vi "beta-2.0.0.vi"() -> ()   [LabVIEW 2016]
uses:
  <vilib>/FPGAPlugInAG/cRIO-9063/niLvFpga_Open_cRIO-9063.vi
  <vilib>/rvi/interface/common/dynamic/niFpgaDynamicAddResources.vi
  <vilib>/Utility/error.llb/Error Cluster From Error Code.vi
  <vilib>/rvi/errors/niLvFpgaAdjustHostInterfaceError.vi
  <vilib>/FPGAPlugInAG/Dynamic/niLvFpga_Close_Dynamic.vi
  <vilib>/rvi/interface/nirviOpenFPGA/nirviOpenFPGA.xnode
  FPGA Bitfiles/multi-functionpr_FPGATarget_multi-function-f_bsn-gyeHrfY.lvbitx
  <vilib>/rvi/interface/nirviReadWriteControl/nirviReadWriteControl.xnode
  <vilib>/rvi/interface/nirviCloseFPGA/nirviCloseFPGA.xnode
  NiFpgaLv.dll
  <vilib>/rvi/interface/Simulation/niFpgaSimulationCallBeginRW.vi
panel:
  in  "OUT15":T1(ring)
  in  "step15":dbl=1.0 format="%#_13g"
  in  "begin15":dbl format="%#_13g"
  in  "end15":dbl=5.0 format="%#_13g"
  in  "OUT14":T1(ring)
  in  "step14":dbl=1.0 format="%#_13g"
  in  "begin14":dbl format="%#_13g"
  in  "end14":dbl=5.0 format="%#_13g"
  in  "OUT13":T1(ring)
  in  "step13":dbl=1.0 format="%#_13g"
  in  "begin13":dbl format="%#_13g"
  in  "end13":dbl=5.0 format="%#_13g"
  in  "OUT12":T1(ring)
  in  "step12":dbl=1.0 format="%#_13g"
  in  "begin12":dbl format="%#_13g"
  in  "end12":dbl=5.0 format="%#_13g"
  in  "OUT11":T1(ring)
  in  "step11":dbl=1.0 format="%#_13g"
  in  "begin11":dbl format="%#_13g"
  in  "end11":dbl=5.0 format="%#_13g"
  in  "OUT10":T1(ring)
  in  "step10":dbl=1.0 format="%#_13g"
  in  "begin10":dbl format="%#_13g"
  in  "end10":dbl=5.0 format="%#_13g"
  in  "OUT9":T1(ring)
  in  "step9":dbl=1.0 format="%#_13g"
  in  "begin9":dbl format="%#_13g"
  in  "end9":dbl=5.0 format="%#_13g"
  in  "OUT8":T1(ring)
  in  "step8":dbl=1.0 format="%#_13g"
  in  "begin8":dbl format="%#_13g"
  in  "end8":dbl=5.0 format="%#_13g"
  in  "OUT7":T1(ring)
  in  "step7":dbl=1.0 format="%#_13g"
  in  "begin7":dbl format="%#_13g"
  in  "end7":dbl=5.0 format="%#_13g"
  in  "OUT6":T1(ring)
  in  "step6":dbl=1.0 format="%#_13g"
  in  "begin6":dbl format="%#_13g"
  in  "end6":dbl=5.0 format="%#_13g"
  in  "OUT5":T1(ring)
  in  "step5":dbl=1.0 format="%#_13g"
  in  "begin5":dbl format="%#_13g"
  in  "end5":dbl=5.0 format="%#_13g"
  in  "OUT4":T1(ring)
  in  "step4":dbl=1.0 format="%#_13g"
  in  "begin4":dbl format="%#_13g"
  in  "end4":dbl=5.0 format="%#_13g"
  in  "OUT3":T1(ring)
  in  "step3":dbl=1.0 format="%#_13g"
  in  "begin3":dbl format="%#_13g"
  in  "end3":dbl=5.0 format="%#_13g"
  in  "OUT2":T1(ring)
  in  "step2":dbl=1.0 format="%#_13g"
  in  "begin2":dbl format="%#_13g"
  in  "end2":dbl=5.0 format="%#_13g"
  in  "OUT1":T1(ring)
  in  "step1":dbl=1.0 format="%#_13g"
  in  "begin1":dbl format="%#_13g"
  in  "end1":dbl=5.0 format="%#_13g"
  in  "end0":dbl=5.0 format="%#_13g"
  in  "begin0":dbl format="%#_13g"
  in  "step0":dbl=1.0 format="%#_13g"
  in  "OUT0":T1(ring)
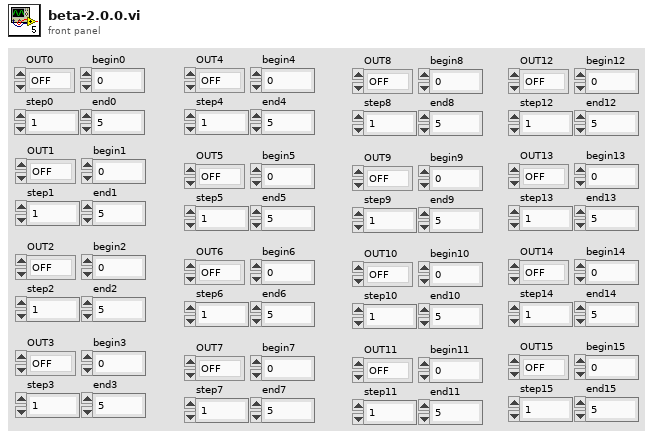
[diagram p1: front panel]
types:
  T1 = enum16{"OFF", "SWITCH", "AND GATE", "OR GATE", "ITERATION"}
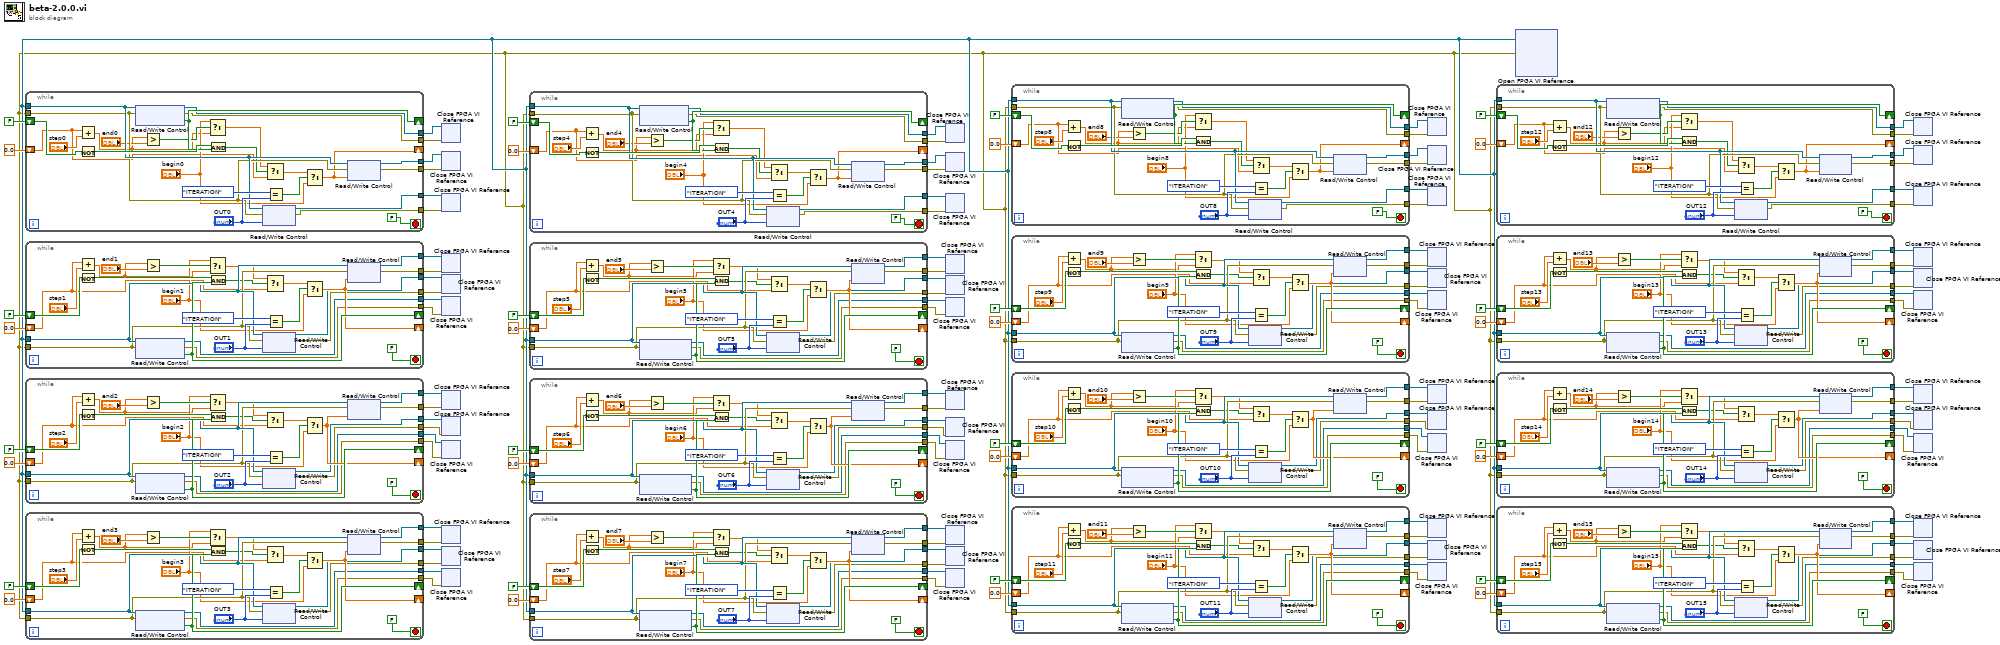
[diagram p0: block diagram]
diagram:
  n1 = xnode "Open FPGA VI Reference"() -> ("FPGA VI Reference Out"=w2:refnum<k20>, "error out"=w1:errorcluster)  [unwired: 2 in]
  n2 = while {
    tunnel: w2 -> [w149]
    tunnel: w1 -> [w148]
    shift-right: [w151] -> _
    shift-left: FALSE -> [w153]
    shift-right: [w146] -> _
    shift-left: 0.0 -> [w138]
    tunnel: [w136] -> w128
    tunnel: [w135] -> w127
    tunnel: [w134] -> w126
    tunnel: [w133] -> w125
    tunnel: [w132] -> w124
    tunnel: [w131] -> w123
    stop <- FALSE stop-if-true
    n3 = Add(x=w138, y="step0") -> (x+y=w140:dbl)
    n4 = Not(x=w153) -> (.not. x?=w152:bool)
    n5 = xnode "Read/Write Control"("FPGA VI Reference In"=w149, "error in"=w148) -> ("FPGA VI Reference Out"=w136:refnum<k20>, "error out"=w135:errorcluster, "Mod2/DIO0"=w151:bool)
    n6 = Greater?(x=w140, y="end0") -> (0:w142:bool)
    n7 = Select(t="begin0", s=w142, f=w140) -> (s? t:f=w139:dbl)
    n8 = And(x=w152, y=w151) -> (x .and. y?=w144:bool)
    n9 = xnode "Read/Write Control"("FPGA VI Reference In"=w149, "error in"=w148, "OUT0"="OUT0") -> ("FPGA VI Reference Out"=w134:refnum<k20>, "error out"=w133:errorcluster)
    n10 = Select(t=w139, s=w144, f=w138) -> (s? t:f=w137:dbl)
    n11 = Equal?(x=T1."ITERATION" ("OUT0"), y="OUT0") -> (x = y?=w147:bool)
    n12 = Select(t=w137, s=w147, f="begin0") -> (s? t:f=w146:dbl)
    n13 = xnode "Read/Write Control"("FPGA VI Reference In"=w149, "error in"=w148, "iter0"=w146) -> ("FPGA VI Reference Out"=w132:refnum<k20>, "error out"=w131:errorcluster)
  }
  n14 = while {
    tunnel: w2 -> [w174]
    tunnel: w1 -> [w173]
    shift-right: [w176] -> _
    shift-left: FALSE -> [w178]
    shift-right: [w171] -> _
    shift-left: 0.0 -> [w163]
    tunnel: [w161] -> w120
    tunnel: [w160] -> w119
    tunnel: [w159] -> w118
    tunnel: [w158] -> w117
    tunnel: [w157] -> w116
    tunnel: [w156] -> w115
    stop <- FALSE stop-if-true
    n15 = Add(x=w163, y="step1") -> (x+y=w165:dbl)
    n16 = Not(x=w178) -> (.not. x?=w177:bool)
    n17 = xnode "Read/Write Control"("FPGA VI Reference In"=w174, "error in"=w173) -> ("FPGA VI Reference Out"=w161:refnum<k20>, "error out"=w160:errorcluster, "Mod2/DIO2"=w176:bool)
    n18 = Greater?(x=w165, y="end1") -> (0:w167:bool)
    n19 = Select(t="begin1", s=w167, f=w165) -> (s? t:f=w164:dbl)
    n20 = And(x=w177, y=w176) -> (x .and. y?=w169:bool)
    n21 = xnode "Read/Write Control"("FPGA VI Reference In"=w174, "error in"=w173, "OUT1"="OUT1") -> ("FPGA VI Reference Out"=w159:refnum<k20>, "error out"=w158:errorcluster)
    n22 = Select(t=w164, s=w169, f=w163) -> (s? t:f=w162:dbl)
    n23 = Equal?(x=T1."ITERATION" ("OUT0"), y="OUT1") -> (x = y?=w172:bool)
    n24 = Select(t=w162, s=w172, f="begin1") -> (s? t:f=w171:dbl)
    n25 = xnode "Read/Write Control"("FPGA VI Reference In"=w174, "error in"=w173, "iter1"=w171) -> ("FPGA VI Reference Out"=w157:refnum<k20>, "error out"=w156:errorcluster)
  }
  n26 = while {
    tunnel: w2 -> [w199]
    tunnel: w1 -> [w198]
    shift-right: [w201] -> _
    shift-left: FALSE -> [w203]
    shift-right: [w196] -> _
    shift-left: 0.0 -> [w188]
    tunnel: [w186] -> w112
    tunnel: [w185] -> w111
    tunnel: [w184] -> w110
    tunnel: [w183] -> w109
    tunnel: [w182] -> w108
    tunnel: [w181] -> w107
    stop <- FALSE stop-if-true
    n27 = Add(x=w188, y="step2") -> (x+y=w190:dbl)
    n28 = Not(x=w203) -> (.not. x?=w202:bool)
    n29 = xnode "Read/Write Control"("FPGA VI Reference In"=w199, "error in"=w198) -> ("FPGA VI Reference Out"=w186:refnum<k20>, "error out"=w185:errorcluster, "Mod2/DIO4"=w201:bool)
    n30 = Greater?(x=w190, y="end2") -> (0:w192:bool)
    n31 = Select(t="begin2", s=w192, f=w190) -> (s? t:f=w189:dbl)
    n32 = And(x=w202, y=w201) -> (x .and. y?=w194:bool)
    n33 = xnode "Read/Write Control"("FPGA VI Reference In"=w199, "error in"=w198, "OUT2"="OUT2") -> ("FPGA VI Reference Out"=w184:refnum<k20>, "error out"=w183:errorcluster)
    n34 = Select(t=w189, s=w194, f=w188) -> (s? t:f=w187:dbl)
    n35 = Equal?(x=T1."ITERATION" ("OUT0"), y="OUT2") -> (x = y?=w197:bool)
    n36 = Select(t=w187, s=w197, f="begin2") -> (s? t:f=w196:dbl)
    n37 = xnode "Read/Write Control"("FPGA VI Reference In"=w199, "error in"=w198, "iter3"=w196) -> ("FPGA VI Reference Out"=w182:refnum<k20>, "error out"=w181:errorcluster)
  }
  n38 = while {
    tunnel: w2 -> [w224]
    tunnel: w1 -> [w223]
    shift-right: [w226] -> _
    shift-left: FALSE -> [w228]
    shift-right: [w221] -> _
    shift-left: 0.0 -> [w213]
    tunnel: [w211] -> w104
    tunnel: [w210] -> w103
    tunnel: [w209] -> w102
    tunnel: [w208] -> w101
    tunnel: [w207] -> w100
    tunnel: [w206] -> w99
    stop <- FALSE stop-if-true
    n39 = Add(x=w213, y="step3") -> (x+y=w215:dbl)
    n40 = Not(x=w228) -> (.not. x?=w227:bool)
    n41 = xnode "Read/Write Control"("FPGA VI Reference In"=w224, "error in"=w223) -> ("FPGA VI Reference Out"=w211:refnum<k20>, "error out"=w210:errorcluster, "Mod2/DIO6"=w226:bool)
    n42 = Greater?(x=w215, y="end3") -> (0:w217:bool)
    n43 = Select(t="begin3", s=w217, f=w215) -> (s? t:f=w214:dbl)
    n44 = And(x=w227, y=w226) -> (x .and. y?=w219:bool)
    n45 = xnode "Read/Write Control"("FPGA VI Reference In"=w224, "error in"=w223, "OUT3"="OUT3") -> ("FPGA VI Reference Out"=w209:refnum<k20>, "error out"=w208:errorcluster)
    n46 = Select(t=w214, s=w219, f=w213) -> (s? t:f=w212:dbl)
    n47 = Equal?(x=T1."ITERATION" ("OUT0"), y="OUT3") -> (x = y?=w222:bool)
    n48 = Select(t=w212, s=w222, f="begin3") -> (s? t:f=w221:dbl)
    n49 = xnode "Read/Write Control"("FPGA VI Reference In"=w224, "error in"=w223, "iter1"=w221) -> ("FPGA VI Reference Out"=w207:refnum<k20>, "error out"=w206:errorcluster)
  }
  n50 = xnode "Close FPGA VI Reference"("FPGA VI Reference In"=w128, "error in"=w127) -> ()  [unwired: 1 out]
  n51 = xnode "Close FPGA VI Reference"("FPGA VI Reference In"=w124, "error in"=w123) -> ()  [unwired: 1 out]
  n52 = xnode "Close FPGA VI Reference"("FPGA VI Reference In"=w126, "error in"=w125) -> ()  [unwired: 1 out]
  n53 = xnode "Close FPGA VI Reference"("FPGA VI Reference In"=w116, "error in"=w115) -> ()  [unwired: 1 out]
  n54 = xnode "Close FPGA VI Reference"("FPGA VI Reference In"=w118, "error in"=w117) -> ()  [unwired: 1 out]
  n55 = xnode "Close FPGA VI Reference"("FPGA VI Reference In"=w120, "error in"=w119) -> ()  [unwired: 1 out]
  n56 = xnode "Close FPGA VI Reference"("FPGA VI Reference In"=w108, "error in"=w107) -> ()  [unwired: 1 out]
  n57 = xnode "Close FPGA VI Reference"("FPGA VI Reference In"=w110, "error in"=w109) -> ()  [unwired: 1 out]
  n58 = xnode "Close FPGA VI Reference"("FPGA VI Reference In"=w112, "error in"=w111) -> ()  [unwired: 1 out]
  n59 = xnode "Close FPGA VI Reference"("FPGA VI Reference In"=w100, "error in"=w99) -> ()  [unwired: 1 out]
  n60 = xnode "Close FPGA VI Reference"("FPGA VI Reference In"=w102, "error in"=w101) -> ()  [unwired: 1 out]
  n61 = xnode "Close FPGA VI Reference"("FPGA VI Reference In"=w104, "error in"=w103) -> ()  [unwired: 1 out]
  n62 = while {
    tunnel: w2 -> [w249]
    tunnel: w1 -> [w248]
    shift-right: [w251] -> _
    shift-left: FALSE -> [w253]
    shift-right: [w246] -> _
    shift-left: 0.0 -> [w238]
    tunnel: [w236] -> w96
    tunnel: [w235] -> w95
    tunnel: [w234] -> w94
    tunnel: [w233] -> w93
    tunnel: [w232] -> w92
    tunnel: [w231] -> w91
    stop <- FALSE stop-if-true
    n63 = Add(x=w238, y="step4") -> (x+y=w240:dbl)
    n64 = Not(x=w253) -> (.not. x?=w252:bool)
    n65 = xnode "Read/Write Control"("FPGA VI Reference In"=w249, "error in"=w248) -> ("FPGA VI Reference Out"=w236:refnum<k20>, "error out"=w235:errorcluster, "Mod2/DIO8"=w251:bool)
    n66 = Greater?(x=w240, y="end4") -> (0:w242:bool)
    n67 = Select(t="begin4", s=w242, f=w240) -> (s? t:f=w239:dbl)
    n68 = And(x=w252, y=w251) -> (x .and. y?=w244:bool)
    n69 = xnode "Read/Write Control"("FPGA VI Reference In"=w249, "error in"=w248, "OUT4"="OUT4") -> ("FPGA VI Reference Out"=w234:refnum<k20>, "error out"=w233:errorcluster)
    n70 = Select(t=w239, s=w244, f=w238) -> (s? t:f=w237:dbl)
    n71 = Equal?(x=T1."ITERATION" ("OUT0"), y="OUT4") -> (x = y?=w247:bool)
    n72 = Select(t=w237, s=w247, f="begin4") -> (s? t:f=w246:dbl)
    n73 = xnode "Read/Write Control"("FPGA VI Reference In"=w249, "error in"=w248, "iter4"=w246) -> ("FPGA VI Reference Out"=w232:refnum<k20>, "error out"=w231:errorcluster)
  }
  n74 = while {
    tunnel: w2 -> [w274]
    tunnel: w1 -> [w273]
    shift-right: [w276] -> _
    shift-left: FALSE -> [w278]
    shift-right: [w271] -> _
    shift-left: 0.0 -> [w263]
    tunnel: [w261] -> w88
    tunnel: [w260] -> w87
    tunnel: [w259] -> w86
    tunnel: [w258] -> w85
    tunnel: [w257] -> w84
    tunnel: [w256] -> w83
    stop <- FALSE stop-if-true
    n75 = Add(x=w263, y="step5") -> (x+y=w265:dbl)
    n76 = Not(x=w278) -> (.not. x?=w277:bool)
    n77 = xnode "Read/Write Control"("FPGA VI Reference In"=w274, "error in"=w273) -> ("FPGA VI Reference Out"=w261:refnum<k20>, "error out"=w260:errorcluster, "Mod2/DIO10"=w276:bool)
    n78 = Greater?(x=w265, y="end5") -> (0:w267:bool)
    n79 = Select(t="begin5", s=w267, f=w265) -> (s? t:f=w264:dbl)
    n80 = And(x=w277, y=w276) -> (x .and. y?=w269:bool)
    n81 = xnode "Read/Write Control"("FPGA VI Reference In"=w274, "error in"=w273, "OUT5"="OUT5") -> ("FPGA VI Reference Out"=w259:refnum<k20>, "error out"=w258:errorcluster)
    n82 = Select(t=w264, s=w269, f=w263) -> (s? t:f=w262:dbl)
    n83 = Equal?(x=T1."ITERATION" ("OUT0"), y="OUT5") -> (x = y?=w272:bool)
    n84 = Select(t=w262, s=w272, f="begin5") -> (s? t:f=w271:dbl)
    n85 = xnode "Read/Write Control"("FPGA VI Reference In"=w274, "error in"=w273, "iter5"=w271) -> ("FPGA VI Reference Out"=w257:refnum<k20>, "error out"=w256:errorcluster)
  }
  n86 = while {
    tunnel: w2 -> [w299]
    tunnel: w1 -> [w298]
    shift-right: [w301] -> _
    shift-left: FALSE -> [w303]
    shift-right: [w296] -> _
    shift-left: 0.0 -> [w288]
    tunnel: [w286] -> w80
    tunnel: [w285] -> w79
    tunnel: [w284] -> w78
    tunnel: [w283] -> w77
    tunnel: [w282] -> w76
    tunnel: [w281] -> w75
    stop <- FALSE stop-if-true
    n87 = Add(x=w288, y="step6") -> (x+y=w290:dbl)
    n88 = Not(x=w303) -> (.not. x?=w302:bool)
    n89 = xnode "Read/Write Control"("FPGA VI Reference In"=w299, "error in"=w298) -> ("FPGA VI Reference Out"=w286:refnum<k20>, "error out"=w285:errorcluster, "Mod2/DIO12"=w301:bool)
    n90 = Greater?(x=w290, y="end6") -> (0:w292:bool)
    n91 = Select(t="begin6", s=w292, f=w290) -> (s? t:f=w289:dbl)
    n92 = And(x=w302, y=w301) -> (x .and. y?=w294:bool)
    n93 = xnode "Read/Write Control"("FPGA VI Reference In"=w299, "error in"=w298, "OUT6"="OUT6") -> ("FPGA VI Reference Out"=w284:refnum<k20>, "error out"=w283:errorcluster)
    n94 = Select(t=w289, s=w294, f=w288) -> (s? t:f=w287:dbl)
    n95 = Equal?(x=T1."ITERATION" ("OUT0"), y="OUT6") -> (x = y?=w297:bool)
    n96 = Select(t=w287, s=w297, f="begin6") -> (s? t:f=w296:dbl)
    n97 = xnode "Read/Write Control"("FPGA VI Reference In"=w299, "error in"=w298, "iter6"=w296) -> ("FPGA VI Reference Out"=w282:refnum<k20>, "error out"=w281:errorcluster)
  }
  n98 = while {
    tunnel: w2 -> [w324]
    tunnel: w1 -> [w323]
    shift-right: [w326] -> _
    shift-left: FALSE -> [w328]
    shift-right: [w321] -> _
    shift-left: 0.0 -> [w313]
    tunnel: [w311] -> w72
    tunnel: [w310] -> w71
    tunnel: [w309] -> w70
    tunnel: [w308] -> w69
    tunnel: [w307] -> w68
    tunnel: [w306] -> w67
    stop <- FALSE stop-if-true
    n99 = Add(x=w313, y="step7") -> (x+y=w315:dbl)
    n100 = Not(x=w328) -> (.not. x?=w327:bool)
    n101 = xnode "Read/Write Control"("FPGA VI Reference In"=w324, "error in"=w323) -> ("FPGA VI Reference Out"=w311:refnum<k20>, "error out"=w310:errorcluster, "Mod2/DIO14"=w326:bool)
    n102 = Greater?(x=w315, y="end7") -> (0:w317:bool)
    n103 = Select(t="begin7", s=w317, f=w315) -> (s? t:f=w314:dbl)
    n104 = And(x=w327, y=w326) -> (x .and. y?=w319:bool)
    n105 = xnode "Read/Write Control"("FPGA VI Reference In"=w324, "error in"=w323, "OUT7"="OUT7") -> ("FPGA VI Reference Out"=w309:refnum<k20>, "error out"=w308:errorcluster)
    n106 = Select(t=w314, s=w319, f=w313) -> (s? t:f=w312:dbl)
    n107 = Equal?(x=T1."ITERATION" ("OUT0"), y="OUT7") -> (x = y?=w322:bool)
    n108 = Select(t=w312, s=w322, f="begin7") -> (s? t:f=w321:dbl)
    n109 = xnode "Read/Write Control"("FPGA VI Reference In"=w324, "error in"=w323, "iter7"=w321) -> ("FPGA VI Reference Out"=w307:refnum<k20>, "error out"=w306:errorcluster)
  }
  n110 = xnode "Close FPGA VI Reference"("FPGA VI Reference In"=w96, "error in"=w95) -> ()  [unwired: 1 out]
  n111 = xnode "Close FPGA VI Reference"("FPGA VI Reference In"=w92, "error in"=w91) -> ()  [unwired: 1 out]
  n112 = xnode "Close FPGA VI Reference"("FPGA VI Reference In"=w94, "error in"=w93) -> ()  [unwired: 1 out]
  n113 = xnode "Close FPGA VI Reference"("FPGA VI Reference In"=w84, "error in"=w83) -> ()  [unwired: 1 out]
  n114 = xnode "Close FPGA VI Reference"("FPGA VI Reference In"=w86, "error in"=w85) -> ()  [unwired: 1 out]
  n115 = xnode "Close FPGA VI Reference"("FPGA VI Reference In"=w88, "error in"=w87) -> ()  [unwired: 1 out]
  n116 = xnode "Close FPGA VI Reference"("FPGA VI Reference In"=w76, "error in"=w75) -> ()  [unwired: 1 out]
  n117 = xnode "Close FPGA VI Reference"("FPGA VI Reference In"=w78, "error in"=w77) -> ()  [unwired: 1 out]
  n118 = xnode "Close FPGA VI Reference"("FPGA VI Reference In"=w80, "error in"=w79) -> ()  [unwired: 1 out]
  n119 = xnode "Close FPGA VI Reference"("FPGA VI Reference In"=w68, "error in"=w67) -> ()  [unwired: 1 out]
  n120 = xnode "Close FPGA VI Reference"("FPGA VI Reference In"=w70, "error in"=w69) -> ()  [unwired: 1 out]
  n121 = xnode "Close FPGA VI Reference"("FPGA VI Reference In"=w72, "error in"=w71) -> ()  [unwired: 1 out]
  n122 = while {
    tunnel: w2 -> [w349]
    tunnel: w1 -> [w348]
    shift-right: [w351] -> _
    shift-left: FALSE -> [w353]
    shift-right: [w346] -> _
    shift-left: 0.0 -> [w338]
    tunnel: [w336] -> w64
    tunnel: [w335] -> w63
    tunnel: [w334] -> w62
    tunnel: [w333] -> w61
    tunnel: [w332] -> w60
    tunnel: [w331] -> w59
    stop <- FALSE stop-if-true
    n123 = Add(x=w338, y="step8") -> (x+y=w340:dbl)
    n124 = Not(x=w353) -> (.not. x?=w352:bool)
    n125 = xnode "Read/Write Control"("FPGA VI Reference In"=w349, "error in"=w348) -> ("FPGA VI Reference Out"=w336:refnum<k20>, "error out"=w335:errorcluster, "Mod2/DIO16"=w351:bool)
    n126 = Greater?(x=w340, y="end8") -> (0:w342:bool)
    n127 = Select(t="begin8", s=w342, f=w340) -> (s? t:f=w339:dbl)
    n128 = And(x=w352, y=w351) -> (x .and. y?=w344:bool)
    n129 = xnode "Read/Write Control"("FPGA VI Reference In"=w349, "error in"=w348, "OUT8"="OUT8") -> ("FPGA VI Reference Out"=w334:refnum<k20>, "error out"=w333:errorcluster)
    n130 = Select(t=w339, s=w344, f=w338) -> (s? t:f=w337:dbl)
    n131 = Equal?(x=T1."ITERATION" ("OUT0"), y="OUT8") -> (x = y?=w347:bool)
    n132 = Select(t=w337, s=w347, f="begin8") -> (s? t:f=w346:dbl)
    n133 = xnode "Read/Write Control"("FPGA VI Reference In"=w349, "error in"=w348, "iter8"=w346) -> ("FPGA VI Reference Out"=w332:refnum<k20>, "error out"=w331:errorcluster)
  }
  n134 = while {
    tunnel: w2 -> [w374]
    tunnel: w1 -> [w373]
    shift-right: [w376] -> _
    shift-left: FALSE -> [w378]
    shift-right: [w371] -> _
    shift-left: 0.0 -> [w363]
    tunnel: [w361] -> w56
    tunnel: [w360] -> w55
    tunnel: [w359] -> w54
    tunnel: [w358] -> w53
    tunnel: [w357] -> w52
    tunnel: [w356] -> w51
    stop <- FALSE stop-if-true
    n135 = Add(x=w363, y="step9") -> (x+y=w365:dbl)
    n136 = Not(x=w378) -> (.not. x?=w377:bool)
    n137 = xnode "Read/Write Control"("FPGA VI Reference In"=w374, "error in"=w373) -> ("FPGA VI Reference Out"=w361:refnum<k20>, "error out"=w360:errorcluster, "Mod2/DIO18"=w376:bool)
    n138 = Greater?(x=w365, y="end9") -> (0:w367:bool)
    n139 = Select(t="begin9", s=w367, f=w365) -> (s? t:f=w364:dbl)
    n140 = And(x=w377, y=w376) -> (x .and. y?=w369:bool)
    n141 = xnode "Read/Write Control"("FPGA VI Reference In"=w374, "error in"=w373, "OUT9"="OUT9") -> ("FPGA VI Reference Out"=w359:refnum<k20>, "error out"=w358:errorcluster)
    n142 = Select(t=w364, s=w369, f=w363) -> (s? t:f=w362:dbl)
    n143 = Equal?(x=T1."ITERATION" ("OUT0"), y="OUT9") -> (x = y?=w372:bool)
    n144 = Select(t=w362, s=w372, f="begin9") -> (s? t:f=w371:dbl)
    n145 = xnode "Read/Write Control"("FPGA VI Reference In"=w374, "error in"=w373, "iter9"=w371) -> ("FPGA VI Reference Out"=w357:refnum<k20>, "error out"=w356:errorcluster)
  }
  n146 = while {
    tunnel: w2 -> [w399]
    tunnel: w1 -> [w398]
    shift-right: [w401] -> _
    shift-left: FALSE -> [w403]
    shift-right: [w396] -> _
    shift-left: 0.0 -> [w388]
    tunnel: [w386] -> w48
    tunnel: [w385] -> w47
    tunnel: [w384] -> w46
    tunnel: [w383] -> w45
    tunnel: [w382] -> w44
    tunnel: [w381] -> w43
    stop <- FALSE stop-if-true
    n147 = Add(x=w388, y="step10") -> (x+y=w390:dbl)
    n148 = Not(x=w403) -> (.not. x?=w402:bool)
    n149 = xnode "Read/Write Control"("FPGA VI Reference In"=w399, "error in"=w398) -> ("FPGA VI Reference Out"=w386:refnum<k20>, "error out"=w385:errorcluster, "Mod2/DIO20"=w401:bool)
    n150 = Greater?(x=w390, y="end10") -> (0:w392:bool)
    n151 = Select(t="begin10", s=w392, f=w390) -> (s? t:f=w389:dbl)
    n152 = And(x=w402, y=w401) -> (x .and. y?=w394:bool)
    n153 = xnode "Read/Write Control"("FPGA VI Reference In"=w399, "error in"=w398, "OUT10"="OUT10") -> ("FPGA VI Reference Out"=w384:refnum<k20>, "error out"=w383:errorcluster)
    n154 = Select(t=w389, s=w394, f=w388) -> (s? t:f=w387:dbl)
    n155 = Equal?(x=T1."ITERATION" ("OUT0"), y="OUT10") -> (x = y?=w397:bool)
    n156 = Select(t=w387, s=w397, f="begin10") -> (s? t:f=w396:dbl)
    n157 = xnode "Read/Write Control"("FPGA VI Reference In"=w399, "error in"=w398, "iter10"=w396) -> ("FPGA VI Reference Out"=w382:refnum<k20>, "error out"=w381:errorcluster)
  }
  n158 = while {
    tunnel: w2 -> [w424]
    tunnel: w1 -> [w423]
    shift-right: [w426] -> _
    shift-left: FALSE -> [w428]
    shift-right: [w421] -> _
    shift-left: 0.0 -> [w413]
    tunnel: [w411] -> w40
    tunnel: [w410] -> w39
    tunnel: [w409] -> w38
    tunnel: [w408] -> w37
    tunnel: [w407] -> w36
    tunnel: [w406] -> w35
    stop <- FALSE stop-if-true
    n159 = Add(x=w413, y="step11") -> (x+y=w415:dbl)
    n160 = Not(x=w428) -> (.not. x?=w427:bool)
    n161 = xnode "Read/Write Control"("FPGA VI Reference In"=w424, "error in"=w423) -> ("FPGA VI Reference Out"=w411:refnum<k20>, "error out"=w410:errorcluster, "Mod2/DIO22"=w426:bool)
    n162 = Greater?(x=w415, y="end11") -> (0:w417:bool)
    n163 = Select(t="begin11", s=w417, f=w415) -> (s? t:f=w414:dbl)
    n164 = And(x=w427, y=w426) -> (x .and. y?=w419:bool)
    n165 = xnode "Read/Write Control"("FPGA VI Reference In"=w424, "error in"=w423, "OUT11"="OUT11") -> ("FPGA VI Reference Out"=w409:refnum<k20>, "error out"=w408:errorcluster)
    n166 = Select(t=w414, s=w419, f=w413) -> (s? t:f=w412:dbl)
    n167 = Equal?(x=T1."ITERATION" ("OUT0"), y="OUT11") -> (x = y?=w422:bool)
    n168 = Select(t=w412, s=w422, f="begin11") -> (s? t:f=w421:dbl)
    n169 = xnode "Read/Write Control"("FPGA VI Reference In"=w424, "error in"=w423, "iter11"=w421) -> ("FPGA VI Reference Out"=w407:refnum<k20>, "error out"=w406:errorcluster)
  }
  n170 = xnode "Close FPGA VI Reference"("FPGA VI Reference In"=w64, "error in"=w63) -> ()  [unwired: 1 out]
  n171 = xnode "Close FPGA VI Reference"("FPGA VI Reference In"=w60, "error in"=w59) -> ()  [unwired: 1 out]
  n172 = xnode "Close FPGA VI Reference"("FPGA VI Reference In"=w62, "error in"=w61) -> ()  [unwired: 1 out]
  n173 = xnode "Close FPGA VI Reference"("FPGA VI Reference In"=w52, "error in"=w51) -> ()  [unwired: 1 out]
  n174 = xnode "Close FPGA VI Reference"("FPGA VI Reference In"=w54, "error in"=w53) -> ()  [unwired: 1 out]
  n175 = xnode "Close FPGA VI Reference"("FPGA VI Reference In"=w56, "error in"=w55) -> ()  [unwired: 1 out]
  n176 = xnode "Close FPGA VI Reference"("FPGA VI Reference In"=w44, "error in"=w43) -> ()  [unwired: 1 out]
  n177 = xnode "Close FPGA VI Reference"("FPGA VI Reference In"=w46, "error in"=w45) -> ()  [unwired: 1 out]
  n178 = xnode "Close FPGA VI Reference"("FPGA VI Reference In"=w48, "error in"=w47) -> ()  [unwired: 1 out]
  n179 = xnode "Close FPGA VI Reference"("FPGA VI Reference In"=w36, "error in"=w35) -> ()  [unwired: 1 out]
  n180 = xnode "Close FPGA VI Reference"("FPGA VI Reference In"=w38, "error in"=w37) -> ()  [unwired: 1 out]
  n181 = xnode "Close FPGA VI Reference"("FPGA VI Reference In"=w40, "error in"=w39) -> ()  [unwired: 1 out]
  n182 = while {
    tunnel: w2 -> [w449]
    tunnel: w1 -> [w448]
    shift-right: [w451] -> _
    shift-left: FALSE -> [w453]
    shift-right: [w446] -> _
    shift-left: 0.0 -> [w438]
    tunnel: [w436] -> w32
    tunnel: [w435] -> w31
    tunnel: [w434] -> w30
    tunnel: [w433] -> w29
    tunnel: [w432] -> w28
    tunnel: [w431] -> w27
    stop <- FALSE stop-if-true
    n183 = Add(x=w438, y="step12") -> (x+y=w440:dbl)
    n184 = Not(x=w453) -> (.not. x?=w452:bool)
    n185 = xnode "Read/Write Control"("FPGA VI Reference In"=w449, "error in"=w448) -> ("FPGA VI Reference Out"=w436:refnum<k20>, "error out"=w435:errorcluster, "Mod2/DIO24"=w451:bool)
    n186 = Greater?(x=w440, y="end12") -> (0:w442:bool)
    n187 = Select(t="begin12", s=w442, f=w440) -> (s? t:f=w439:dbl)
    n188 = And(x=w452, y=w451) -> (x .and. y?=w444:bool)
    n189 = xnode "Read/Write Control"("FPGA VI Reference In"=w449, "error in"=w448, "OUT12"="OUT12") -> ("FPGA VI Reference Out"=w434:refnum<k20>, "error out"=w433:errorcluster)
    n190 = Select(t=w439, s=w444, f=w438) -> (s? t:f=w437:dbl)
    n191 = Equal?(x=T1."ITERATION" ("OUT0"), y="OUT12") -> (x = y?=w447:bool)
    n192 = Select(t=w437, s=w447, f="begin12") -> (s? t:f=w446:dbl)
    n193 = xnode "Read/Write Control"("FPGA VI Reference In"=w449, "error in"=w448, "iter12"=w446) -> ("FPGA VI Reference Out"=w432:refnum<k20>, "error out"=w431:errorcluster)
  }
  n194 = while {
    tunnel: w2 -> [w474]
    tunnel: w1 -> [w473]
    shift-right: [w476] -> _
    shift-left: FALSE -> [w478]
    shift-right: [w471] -> _
    shift-left: 0.0 -> [w463]
    tunnel: [w461] -> w24
    tunnel: [w460] -> w23
    tunnel: [w459] -> w22
    tunnel: [w458] -> w21
    tunnel: [w457] -> w20
    tunnel: [w456] -> w19
    stop <- FALSE stop-if-true
    n195 = Add(x=w463, y="step13") -> (x+y=w465:dbl)
    n196 = Not(x=w478) -> (.not. x?=w477:bool)
    n197 = xnode "Read/Write Control"("FPGA VI Reference In"=w474, "error in"=w473) -> ("FPGA VI Reference Out"=w461:refnum<k20>, "error out"=w460:errorcluster, "Mod2/DIO26"=w476:bool)
    n198 = Greater?(x=w465, y="end13") -> (0:w467:bool)
    n199 = Select(t="begin13", s=w467, f=w465) -> (s? t:f=w464:dbl)
    n200 = And(x=w477, y=w476) -> (x .and. y?=w469:bool)
    n201 = xnode "Read/Write Control"("FPGA VI Reference In"=w474, "error in"=w473, "OUT13"="OUT13") -> ("FPGA VI Reference Out"=w459:refnum<k20>, "error out"=w458:errorcluster)
    n202 = Select(t=w464, s=w469, f=w463) -> (s? t:f=w462:dbl)
    n203 = Equal?(x=T1."ITERATION" ("OUT0"), y="OUT13") -> (x = y?=w472:bool)
    n204 = Select(t=w462, s=w472, f="begin13") -> (s? t:f=w471:dbl)
    n205 = xnode "Read/Write Control"("FPGA VI Reference In"=w474, "error in"=w473, "iter13"=w471) -> ("FPGA VI Reference Out"=w457:refnum<k20>, "error out"=w456:errorcluster)
  }
  n206 = while {
    tunnel: w2 -> [w499]
    tunnel: w1 -> [w498]
    shift-right: [w501] -> _
    shift-left: FALSE -> [w503]
    shift-right: [w496] -> _
    shift-left: 0.0 -> [w488]
    tunnel: [w486] -> w16
    tunnel: [w485] -> w15
    tunnel: [w484] -> w14
    tunnel: [w483] -> w13
    tunnel: [w482] -> w12
    tunnel: [w481] -> w11
    stop <- FALSE stop-if-true
    n207 = Add(x=w488, y="step14") -> (x+y=w490:dbl)
    n208 = Not(x=w503) -> (.not. x?=w502:bool)
    n209 = xnode "Read/Write Control"("FPGA VI Reference In"=w499, "error in"=w498) -> ("FPGA VI Reference Out"=w486:refnum<k20>, "error out"=w485:errorcluster, "Mod2/DIO28"=w501:bool)
    n210 = Greater?(x=w490, y="end14") -> (0:w492:bool)
    n211 = Select(t="begin14", s=w492, f=w490) -> (s? t:f=w489:dbl)
    n212 = And(x=w502, y=w501) -> (x .and. y?=w494:bool)
    n213 = xnode "Read/Write Control"("FPGA VI Reference In"=w499, "error in"=w498, "OUT14"="OUT14") -> ("FPGA VI Reference Out"=w484:refnum<k20>, "error out"=w483:errorcluster)
    n214 = Select(t=w489, s=w494, f=w488) -> (s? t:f=w487:dbl)
    n215 = Equal?(x=T1."ITERATION" ("OUT0"), y="OUT14") -> (x = y?=w497:bool)
    n216 = Select(t=w487, s=w497, f="begin14") -> (s? t:f=w496:dbl)
    n217 = xnode "Read/Write Control"("FPGA VI Reference In"=w499, "error in"=w498, "iter14"=w496) -> ("FPGA VI Reference Out"=w482:refnum<k20>, "error out"=w481:errorcluster)
  }
  n218 = while {
    tunnel: w2 -> [w524]
    tunnel: w1 -> [w523]
    shift-right: [w526] -> _
    shift-left: FALSE -> [w528]
    shift-right: [w521] -> _
    shift-left: 0.0 -> [w513]
    tunnel: [w511] -> w8
    tunnel: [w510] -> w7
    tunnel: [w509] -> w6
    tunnel: [w508] -> w5
    tunnel: [w507] -> w4
    tunnel: [w506] -> w3
    stop <- FALSE stop-if-true
    n219 = Add(x=w513, y="step15") -> (x+y=w515:dbl)
    n220 = Not(x=w528) -> (.not. x?=w527:bool)
    n221 = xnode "Read/Write Control"("FPGA VI Reference In"=w524, "error in"=w523) -> ("FPGA VI Reference Out"=w511:refnum<k20>, "error out"=w510:errorcluster, "Mod2/DIO30"=w526:bool)
    n222 = Greater?(x=w515, y="end15") -> (0:w517:bool)
    n223 = Select(t="begin15", s=w517, f=w515) -> (s? t:f=w514:dbl)
    n224 = And(x=w527, y=w526) -> (x .and. y?=w519:bool)
    n225 = xnode "Read/Write Control"("FPGA VI Reference In"=w524, "error in"=w523, "OUT15"="OUT15") -> ("FPGA VI Reference Out"=w509:refnum<k20>, "error out"=w508:errorcluster)
    n226 = Select(t=w514, s=w519, f=w513) -> (s? t:f=w512:dbl)
    n227 = Equal?(x=T1."ITERATION" ("OUT0"), y="OUT15") -> (x = y?=w522:bool)
    n228 = Select(t=w512, s=w522, f="begin15") -> (s? t:f=w521:dbl)
    n229 = xnode "Read/Write Control"("FPGA VI Reference In"=w524, "error in"=w523, "iter15"=w521) -> ("FPGA VI Reference Out"=w507:refnum<k20>, "error out"=w506:errorcluster)
  }
  n230 = xnode "Close FPGA VI Reference"("FPGA VI Reference In"=w32, "error in"=w31) -> ()  [unwired: 1 out]
  n231 = xnode "Close FPGA VI Reference"("FPGA VI Reference In"=w28, "error in"=w27) -> ()  [unwired: 1 out]
  n232 = xnode "Close FPGA VI Reference"("FPGA VI Reference In"=w30, "error in"=w29) -> ()  [unwired: 1 out]
  n233 = xnode "Close FPGA VI Reference"("FPGA VI Reference In"=w20, "error in"=w19) -> ()  [unwired: 1 out]
  n234 = xnode "Close FPGA VI Reference"("FPGA VI Reference In"=w22, "error in"=w21) -> ()  [unwired: 1 out]
  n235 = xnode "Close FPGA VI Reference"("FPGA VI Reference In"=w24, "error in"=w23) -> ()  [unwired: 1 out]
  n236 = xnode "Close FPGA VI Reference"("FPGA VI Reference In"=w12, "error in"=w11) -> ()  [unwired: 1 out]
  n237 = xnode "Close FPGA VI Reference"("FPGA VI Reference In"=w14, "error in"=w13) -> ()  [unwired: 1 out]
  n238 = xnode "Close FPGA VI Reference"("FPGA VI Reference In"=w16, "error in"=w15) -> ()  [unwired: 1 out]
  n239 = xnode "Close FPGA VI Reference"("FPGA VI Reference In"=w4, "error in"=w3) -> ()  [unwired: 1 out]
  n240 = xnode "Close FPGA VI Reference"("FPGA VI Reference In"=w6, "error in"=w5) -> ()  [unwired: 1 out]
  n241 = xnode "Close FPGA VI Reference"("FPGA VI Reference In"=w8, "error in"=w7) -> ()  [unwired: 1 out]
